vi "StartMessage.vi"(8 "error in (no error)":errorcluster, 11 "AcquistionObject in":refnum<class "AcquistionObject.lvclass">) -> (0 "error out":errorcluster, 3 "AcquistionObject out":refnum<class "AcquistionObject.lvclass">)   [LabVIEW 2010, in "AcquistionObject.lvclass"]
uses:
  AcquistionObject.lvclass
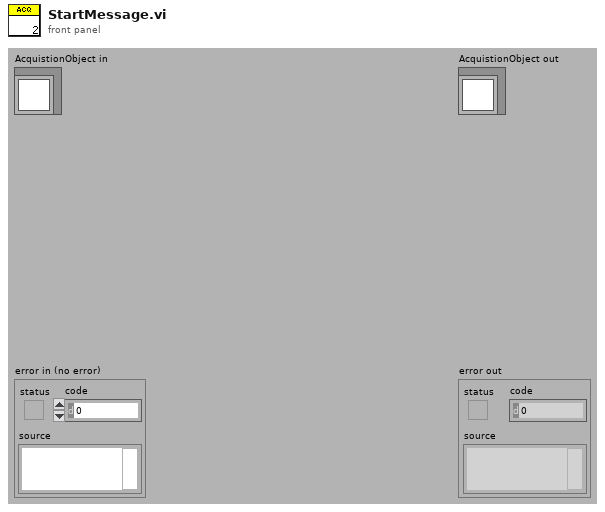
[diagram p1: front panel]
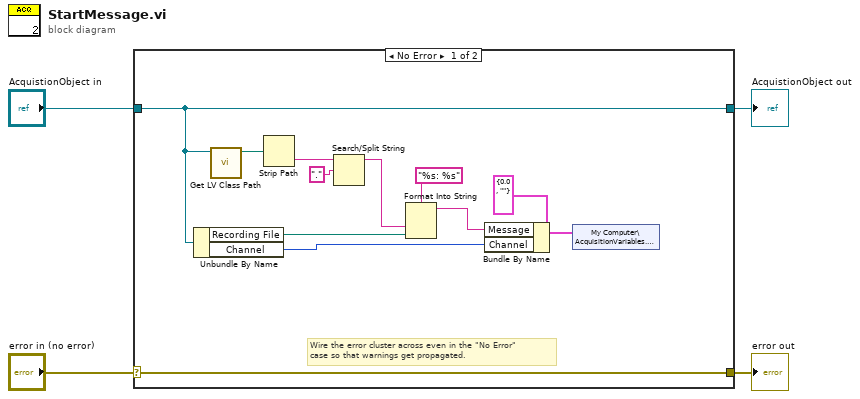
[diagram p0: block diagram]
diagram:
  n1 = case shown="No Error" "error in (no error)" {
    selector: "error in (no error)" -> [w16 w18]
    tunnel: [w16 w18] -> w3
    tunnel: [w9 w17] -> w1
    tunnel: "AcquistionObject in" -> [w9 w17]
    frame No Error {
      # "Wire the error cluster across even in the \"No Error\"\ncase so that warnings get propagated."
      n2 = Unbundle By Name(w9) -> ("Recording File"=w8:path, "Channel"=w11:i16)
      n3 = call <vilib>:"Get LV Class Path.vi"("object"=w9) -> ("class path"=w10:path)  [unwired: 9 in, 1 out]
      n4 = Strip Path(path=w10) -> (name=w6:string)  [unwired: 1 out]
      n5 = Search/Split String(string=w6, search string/char (-)=".") -> (substring before match=w5:string)  [unwired: 1 in, 2 out]
      n6 = Format Into String(format string="%s: %s", w5, w8) -> (resulting string=w12:string)  [unwired: 2 in, 1 out]
      n7 = Bundle By Name(cluster=cluster{"Channel":dbl, "Message":string} {"Channel"=0.0, "Message"=""} ("Message"), "Message"=w12, "Channel"=w11) -> (w15:cluster{"Channel":dbl, "Message":string})
      n8 = shared-variable "My Computer\\AcquisitionVariables.lvlib\\Message"(w15) -> ()  [unwired: 1 in, 1 out]
    }
    frame Error {
    }
  }
  "error out" <- w3
  "AcquistionObject out" <- w1
